vi "CRYInitialize Menu Get.vi"(7 "sAction":string, 8 "Access Level":u16, 9 "Is Disable?":bool, 11 "Main Menu Refnum":refnum<k9>) -> (0 "MenuTFs":bool[](array[boolean]), 1 "MenuTags":string[](array[string])=["VIEW_STEP_SETUP", "VIEW_DATA_VIEW", "VIEW_PROJECT_DOCUMENT", "TOOLS_PAUSE", "TOOLS_START", "TOOLS_STOP", "TOOLS_Continue", "OPERATOR_SIGGEN", "OPERATOR_MULTIMETER", "OPERATOR_OSCILLOSCOPE", "OPERATOR_SPECTRUM", "OPERATOR_RTA", "VIEW_PROJECT", "VIEW_CURVES_LIBRARY"], 2 "MenuNames":string[](array[string])=["Step Setup", "Data View", "Document", "Pause", "Start", "Stop", "Continue", "Signal Generator", "Multimeter", "Oscilloscope", "Spectrum _Analyzer", "RealTime Analyzer", "_Project", "_Curves Library"])   [LabVIEW 2013]
uses:
  CRYProject/CRYProject Editor Global.vi
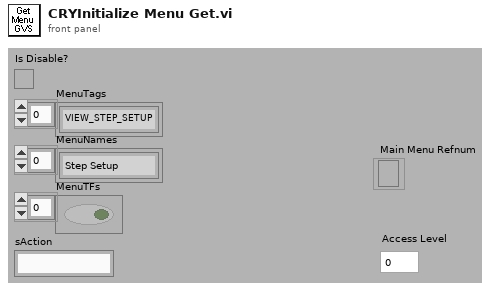
[diagram p1: front panel]
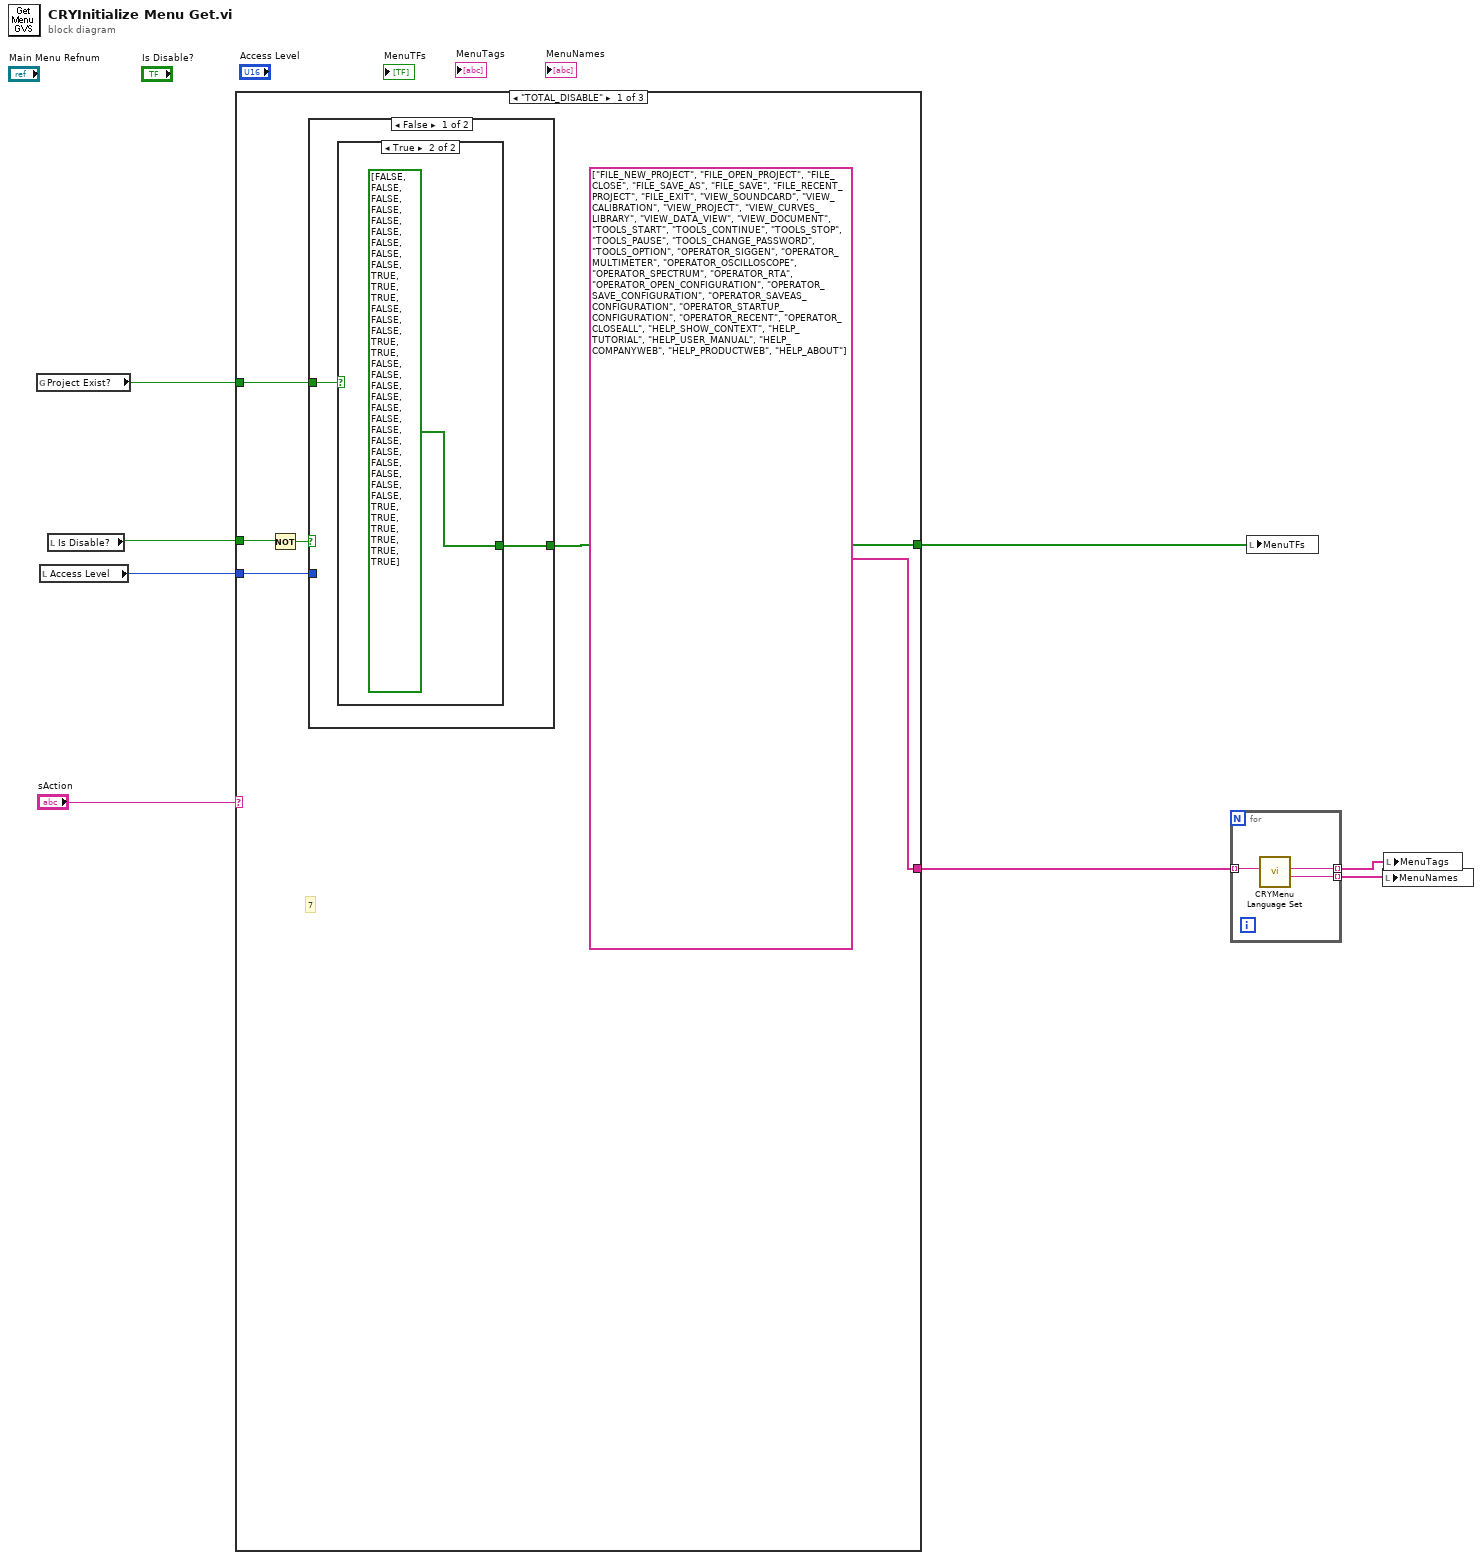
[diagram p0: block diagram]
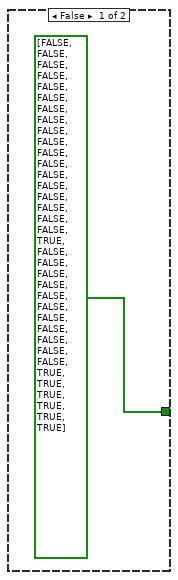
[diagram p2: hidden frame]
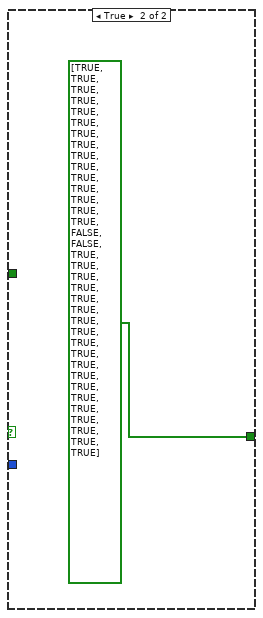
[diagram p3: hidden frame]
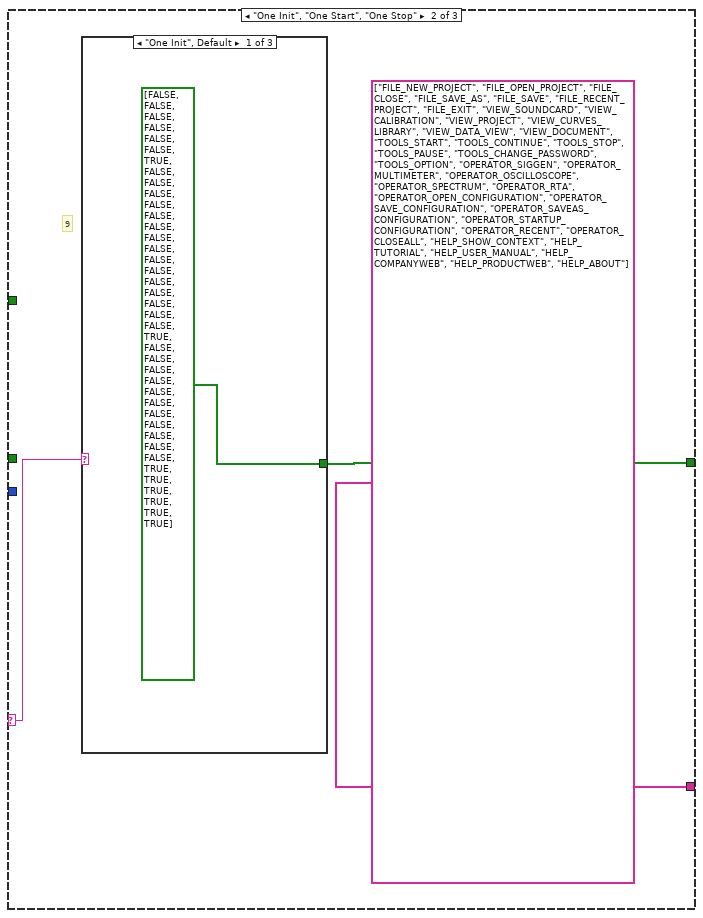
[diagram p4: hidden frame]
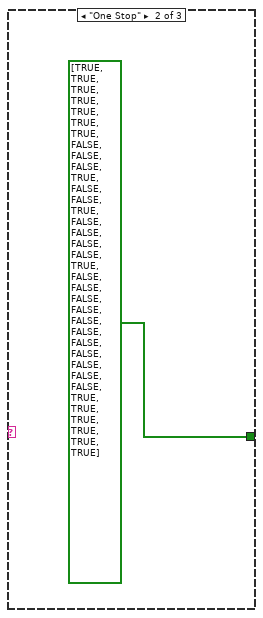
[diagram p5: hidden frame]
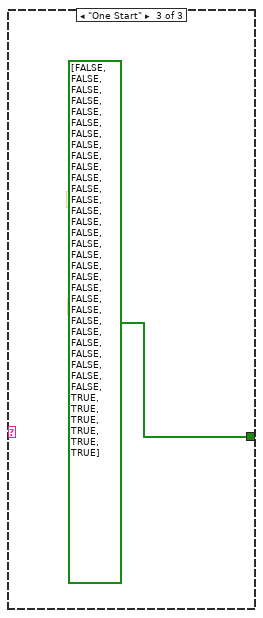
[diagram p6: hidden frame]
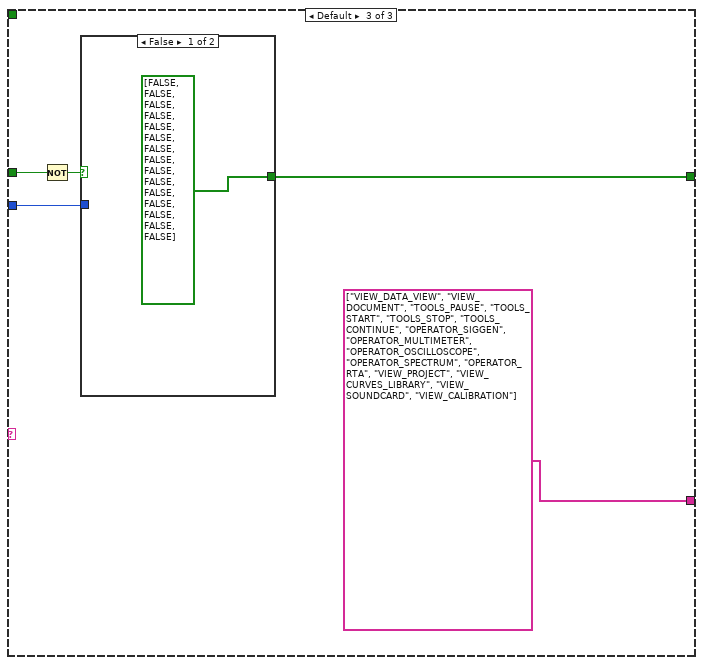
[diagram p7: hidden frame]
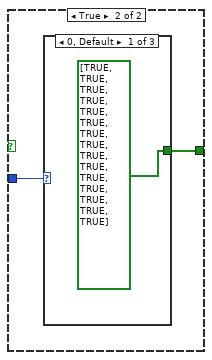
[diagram p8: hidden frame]
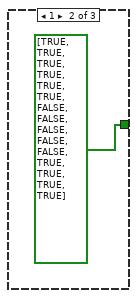
[diagram p9: hidden frame]
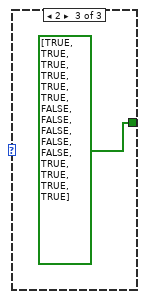
[diagram p10: hidden frame]
diagram:
  n1 = global read "CRYProject Editor Global.vi" "Project Exist?"() -> (w1:bool)
  n2 = local read "Access Level"() -> (w8:u16)
  n3 = local read "Is Disable?"() -> (w7:bool)
  n4 = case shown="\"TOTAL_DISABLE\"" "sAction" {
    selector: "sAction" -> [_ w20 _]
    tunnel: w8 -> [w12 _ w30]
    tunnel: w7 -> [w11 _ w29]
    tunnel: [w10 w21 w27] -> w6
    tunnel: [string[] ["FILE_NEW_PROJECT", "FILE_OPEN_PROJECT", "FILE_CLOSE", "FILE_SAVE_AS", "FILE_SAVE", "FILE_RECENT_PROJECT", "FILE_EXIT", "VIEW_SOUNDCARD", "VIEW_CALIBRATION", "VIEW_PROJECT", "VIEW_CURVES_LIBRARY", "VIEW_DATA_VIEW", "VIEW_DOCUMENT", "TOOLS_START", "TOOLS_CONTINUE", "TOOLS_STOP", "TOOLS_PAUSE", "TOOLS_CHANGE_PASSWORD", "TOOLS_OPTION", "OPERATOR_SIGGEN", "OPERATOR_MULTIMETER", "OPERATOR_OSCILLOSCOPE", "OPERATOR_SPECTRUM", "OPERATOR_RTA", "OPERATOR_OPEN_CONFIGURATION", "OPERATOR_SAVE_CONFIGURATION", "OPERATOR_SAVEAS_CONFIGURATION", "OPERATOR_STARTUP_CONFIGURATION", "OPERATOR_RECENT", "OPERATOR_CLOSEALL", "HELP_SHOW_CONTEXT", "HELP_TUTORIAL", "HELP_USER_MANUAL", "HELP_COMPANYWEB", "HELP_PRODUCTWEB", "HELP_ABOUT"] ("Array") string[] ["FILE_NEW_PROJECT", "FILE_OPEN_PROJECT", "FILE_CLOSE", "FILE_SAVE_AS", "FILE_SAVE", "FILE_RECENT_PROJECT", "FILE_EXIT", "VIEW_SOUNDCARD", "VIEW_CALIBRATION", "VIEW_PROJECT", "VIEW_CURVES_LIBRARY", "VIEW_DATA_VIEW", "VIEW_DOCUMENT", "TOOLS_START", "TOOLS_CONTINUE", "TOOLS_STOP", "TOOLS_PAUSE", "TOOLS_CHANGE_PASSWORD", "TOOLS_OPTION", "OPERATOR_SIGGEN", "OPERATOR_MULTIMETER", "OPERATOR_OSCILLOSCOPE", "OPERATOR_SPECTRUM", "OPERATOR_RTA", "OPERATOR_OPEN_CONFIGURATION", "OPERATOR_SAVE_CONFIGURATION", "OPERATOR_SAVEAS_CONFIGURATION", "OPERATOR_STARTUP_CONFIGURATION", "OPERATOR_RECENT", "OPERATOR_CLOSEALL", "HELP_SHOW_CONTEXT", "HELP_TUTORIAL", "HELP_USER_MANUAL", "HELP_COMPANYWEB", "HELP_PRODUCTWEB", "HELP_ABOUT"] ("Array") string[] ["VIEW_DATA_VIEW", "VIEW_DOCUMENT", "TOOLS_PAUSE", "TOOLS_START", "TOOLS_STOP", "TOOLS_CONTINUE", "OPERATOR_SIGGEN", "OPERATOR_MULTIMETER", "OPERATOR_OSCILLOSCOPE", "OPERATOR_SPECTRUM", "OPERATOR_RTA", "VIEW_PROJECT", "VIEW_CURVES_LIBRARY", "VIEW_SOUNDCARD", "VIEW_CALIBRATION"] ("Array")] -> w5
    tunnel: w1 -> [w9 _ _]
    frame "TOTAL_DISABLE" {
      # "12"
      # "7"
      n5 = Not(x=w11) -> (.not. x?=w14:bool)
      n6 = case shown="False" w14 {
        tunnel: [w16 bool[] [TRUE, TRUE, TRUE, TRUE, TRUE, TRUE, TRUE, TRUE, TRUE, TRUE, TRUE, TRUE, TRUE, TRUE, TRUE, FALSE, FALSE, TRUE, TRUE, TRUE, TRUE, TRUE, TRUE, TRUE, TRUE, TRUE, TRUE, TRUE, TRUE, TRUE, TRUE, TRUE, TRUE, TRUE, TRUE, TRUE]] -> w10
        tunnel: w12 -> [_ _]
        tunnel: w9 -> [w15 _]
        frame False {
          n7 = case shown="True" w15 {
            tunnel: [bool[] [FALSE, FALSE, FALSE, FALSE, FALSE, FALSE, FALSE, FALSE, FALSE, FALSE, FALSE, FALSE, FALSE, FALSE, FALSE, FALSE, FALSE, FALSE, TRUE, FALSE, FALSE, FALSE, FALSE, FALSE, FALSE, FALSE, FALSE, FALSE, FALSE, FALSE, TRUE, TRUE, TRUE, TRUE, TRUE, TRUE] bool[] [FALSE, FALSE, FALSE, FALSE, FALSE, FALSE, FALSE, FALSE, FALSE, TRUE, TRUE, TRUE, FALSE, FALSE, FALSE, TRUE, TRUE, FALSE, FALSE, FALSE, FALSE, FALSE, FALSE, FALSE, FALSE, FALSE, FALSE, FALSE, FALSE, FALSE, TRUE, TRUE, TRUE, TRUE, TRUE, TRUE]] -> w16
            frame False {
            }
            frame True {
            }
          }
        }
        frame True {
          # "12"
          # "17"
        }
      }
    }
    frame "One Init", "One Start", "One Stop" {
      # "9"
      # "17"
      # "9"
      # "6"
      n8 = case shown="\"One Init\", Default" w20 {
        tunnel: [bool[] [FALSE, FALSE, FALSE, FALSE, FALSE, FALSE, TRUE, FALSE, FALSE, FALSE, FALSE, FALSE, FALSE, FALSE, FALSE, FALSE, FALSE, FALSE, FALSE, FALSE, FALSE, FALSE, TRUE, FALSE, FALSE, FALSE, FALSE, FALSE, FALSE, FALSE, FALSE, FALSE, FALSE, FALSE, TRUE, TRUE, TRUE, TRUE, TRUE, TRUE] bool[] [TRUE, TRUE, TRUE, TRUE, TRUE, TRUE, TRUE, FALSE, FALSE, FALSE, TRUE, FALSE, FALSE, TRUE, FALSE, FALSE, FALSE, FALSE, TRUE, FALSE, FALSE, FALSE, FALSE, FALSE, FALSE, FALSE, FALSE, FALSE, FALSE, FALSE, TRUE, TRUE, TRUE, TRUE, TRUE, TRUE] bool[] [FALSE, FALSE, FALSE, FALSE, FALSE, FALSE, FALSE, FALSE, FALSE, FALSE, FALSE, FALSE, FALSE, FALSE, FALSE, FALSE, FALSE, FALSE, FALSE, FALSE, FALSE, FALSE, FALSE, FALSE, FALSE, FALSE, FALSE, FALSE, FALSE, FALSE, TRUE, TRUE, TRUE, TRUE, TRUE, TRUE]] -> w21
        frame "One Init", Default {
          # "6"
        }
        frame "One Stop" {
          # "17"
          # "12"
          # "9"
        }
        frame "One Start" {
          # "9"
          # "17"
        }
      }
    }
    frame Default {
      n9 = Not(x=w29) -> (.not. x?=w28:bool)
      n10 = case shown="False" w28 {
        tunnel: [bool[] [FALSE, FALSE, FALSE, FALSE, FALSE, FALSE, FALSE, FALSE, FALSE, FALSE, FALSE, FALSE, FALSE, FALSE, FALSE] w32] -> w27
        tunnel: w30 -> [_ w33]
        frame False {
        }
        frame True {
          n11 = case shown="0, Default" w33 {
            tunnel: [bool[] [TRUE, TRUE, TRUE, TRUE, TRUE, TRUE, TRUE, TRUE, TRUE, TRUE, TRUE, TRUE, TRUE, TRUE, TRUE] bool[] [TRUE, TRUE, TRUE, TRUE, TRUE, TRUE, FALSE, FALSE, FALSE, FALSE, FALSE, TRUE, TRUE, TRUE, TRUE] bool[] [TRUE, TRUE, TRUE, TRUE, TRUE, TRUE, FALSE, FALSE, FALSE, FALSE, FALSE, TRUE, TRUE, TRUE, TRUE]] -> w32
            frame 0, Default {
            }
            frame 1 {
            }
            frame 2 {
            }
          }
        }
      }
    }
  }
  n12 = for {
    tunnel: w5 -> [w39] mode=indexing
    tunnel: [w38] -> w4 mode=indexing
    tunnel: [w37] -> w2 mode=indexing
    n13 = call "CRYMenu Language Set.vi"("sID"=w39) -> ("sMultibyte_Out"=w37:string, "sID_Out"=w38:string)  [unwired: 7 in, 2 out]
  }
  n14 = local write "MenuTFs"(w6) -> ()
  n15 = local write "MenuNames"(w2) -> ()
  n16 = local write "MenuTags"(w4) -> ()
